vi "TimeShifting.vi"() -> ()   [LabVIEW 2014]
panel:
  in  "Boolean":bool
  out "mag[e^-jwn0.X(w)]":cluster{"-pi to pi":dbl[], dbl[]}(graph)
  out "mag[DTFT{x(n-n0)}]":cluster{"-pi to pi":dbl[], "DTFT op":dbl[]}(graph)
  out "x(n-n0)":dbl[](graph)
  out "x(n)":dbl[](graph)
  out "e^-jwn0.X(w)":cluster{"-pi to pi":dbl[], dbl[]}(graph)
  out "DTFT{x(n-n0)}":cluster{"-pi to pi":dbl[], "DTFT op":dbl[]}(graph)
  out "DTFT{x(n-n0)}":cdb[](array[numeric])
  out "X(w).e^-jwn0":cdb[](array[numeric])
  out "x(n-n0)":dbl[](array[numeric])
  in  "n0":dbl
  out "X(w)":cdb[](array[numeric])
  in  "x(n)":dbl[](array[numeric])
  out "mag response":dbl[](array[numeric])
  # "Instructions"
  # "if\nDTFT{x(n)} ----> X(w)\nthen\nDTFT{x(n-n0)} ----> e^-jwn0.X(w)"
  # "1. enter the input sequence x(n) as array\n2. enter the value by which the time is to be shifted(n>0)\n3. check the input sequence after time shifting\n4. compare the graphs to verify with the property"
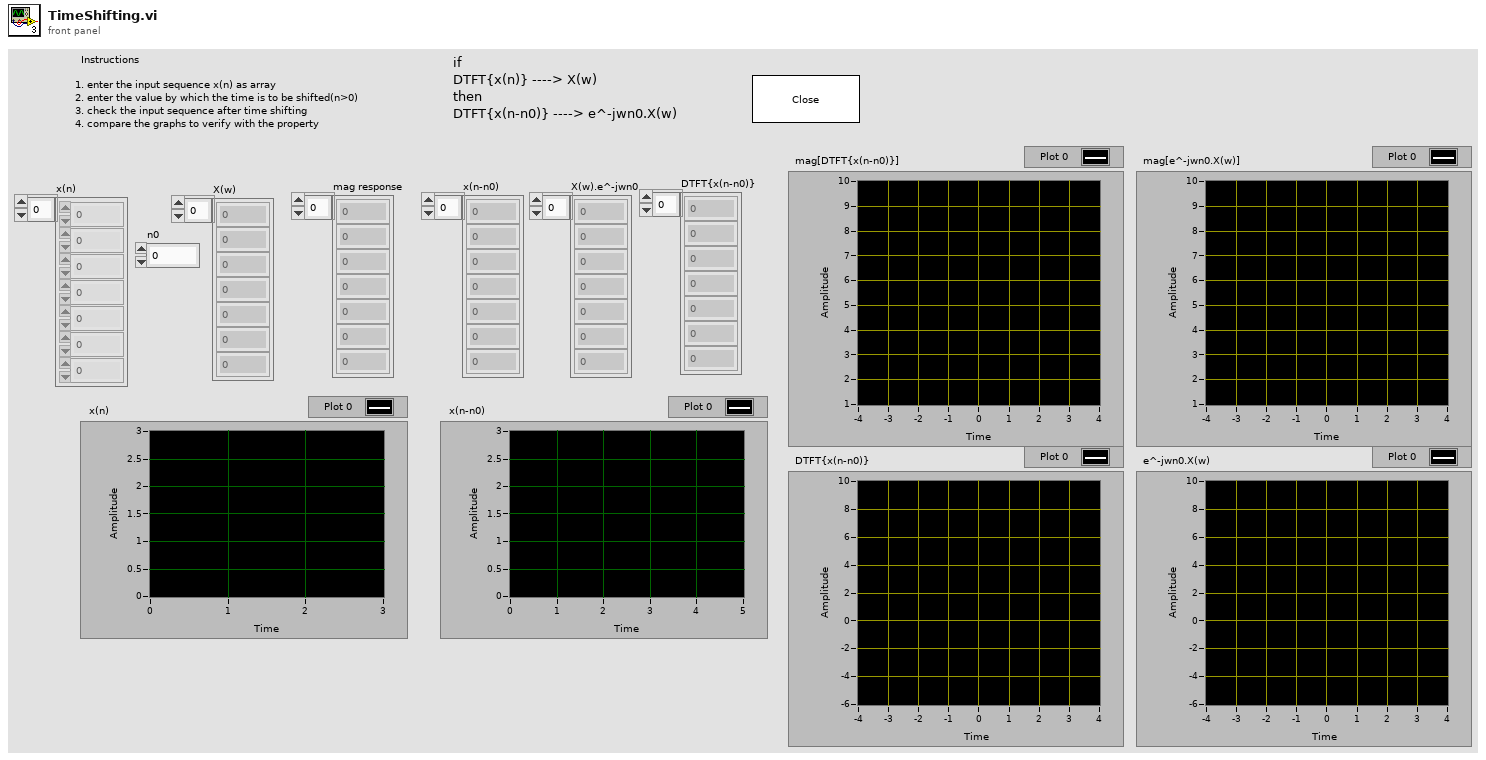
[diagram p1: front panel]
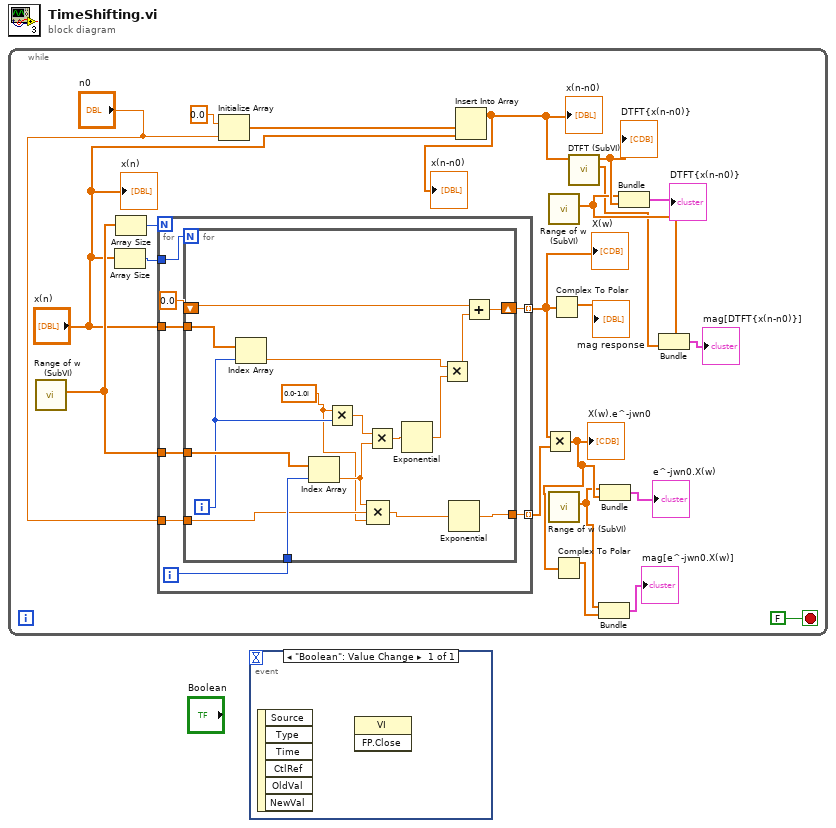
[diagram p0: block diagram]
diagram:
  n1 = while {
    stop <- FALSE stop-if-true
    n2 = call "Range of w (SubVI).vi"() -> ("-pi to pi"=w20:dbl[])  [unwired: 11 in]
    n3 = Array Size(array="x(n)") -> (size(s)=w21:i32)
    n4 = Array Size(array=w20) -> (size(s)=w19:i32)
    n5 = for {
      N: w19 -> [_]
      tunnel: w20 -> [w29]
      tunnel: w21 -> [w28]
      tunnel: "x(n)" -> [w26]
      tunnel: [w25] -> w18 mode=indexing
      tunnel: "n0" -> [w24]
      tunnel: [w23] -> w17 mode=indexing
      i -> [w30]
      n6 = for {
        N: w28 -> [_]
        tunnel: w30 -> [w46]
        tunnel: w29 -> [w45]
        shift-right: [w40] -> w25
        shift-left: 0.0 -> [w39]
        tunnel: w26 -> [w36]
        tunnel: w24 -> [w34]
        tunnel: [w33] -> w23
        i -> [w37]
        w32 = cdb 0.0-1.0i ("x")
        n7 = Index Array(array=w36, index=w37) -> (element=w38:dbl)
        n8 = Index Array(array=w45, index=w46) -> (element=w35:dbl)
        n9 = Multiply(x=w32, y=w37) -> (x*y=w44:cdb)
        n10 = Multiply(x=w44, y=w35) -> (x*y=w43:cdb)
        n11 = Compound Arithmetic op=MULTIPLY(w35, w34, w32) -> (w31:cdb)
        n12 = Exponential(1:w43) -> (0:w42:cdb)
        n13 = Multiply(x=w38, y=w42) -> (x*y=w41:cdb)
        n14 = Exponential(1:w31) -> (0:w33:cdb)
        n15 = Add(x=w39, y=w41) -> (x+y=w40:cdb)
      }
    }
    "X(w)" <- w18
    n16 = Initialize Array(0.0 ("element"), "n0") -> (w11:dbl[])
    n17 = Insert Into Array(array=w11, new element="x(n)") -> (w9:dbl[])  [unwired: 1 in]
    "x(n-n0)" <- w9
    "x(n-n0)" <- w9
    n18 = Multiply(x=w18, y=w17) -> (x*y=w8:cdb[])
    "X(w).e^-jwn0" <- w8
    n19 = call "Range of w (SubVI).vi"() -> ("-pi to pi"=w4:dbl[])  [unwired: 11 in]
    n20 = call "Range of w (SubVI).vi"() -> ("-pi to pi"=w5:dbl[])  [unwired: 11 in]
    n21 = Complex To Polar(r * e^(i*theta)=w18) -> (r=→"mag response":dbl[])  [unwired: 1 out]
    n22 = Complex To Polar(r * e^(i*theta)=w8) -> (r=w7:dbl[])  [unwired: 1 out]
    n23 = call "DTFT (SubVI).vi"("ip array"=w9) -> ("Magnitude op"=w3:dbl[], "DTFT op"=w16:cdb[])  [unwired: 9 in]
    "DTFT{x(n-n0)}" <- w16
    n24 = Bundle("-pi to pi"=w5, w7) -> (→"mag[e^-jwn0.X(w)]":cluster{"-pi to pi":dbl[], dbl[]})  [unwired: 1 in]
    n25 = Bundle("-pi to pi"=w5, w8) -> (→"e^-jwn0.X(w)":cluster{"-pi to pi":dbl[], cdb[]})  [unwired: 1 in]
    n26 = Bundle("-pi to pi"=w4, "DTFT op"=w16) -> (→"DTFT{x(n-n0)}":cluster{"-pi to pi":dbl[], "DTFT op":cdb[]})  [unwired: 1 in]
    n27 = Bundle("-pi to pi"=w4, "Magnitude op"=w3) -> (→"mag[DTFT{x(n-n0)}]":cluster{"-pi to pi":dbl[], "Magnitude op":dbl[]})  [unwired: 1 in]
    "x(n)" <- "x(n)"
  }
  n28 = event shown="[0] \"Boolean\": Value Change" {
    selector: _ -> [_]
    dyn-events: _ -> [_]
    timeout: _ -> [_]
    event "Boolean": Value Change {
      n29 = event-data() -> ()  [unwired: 1 in, 6 out]
      n30 = invoke class="VI" method="FP.Close"() -> ()  [unwired: 3 in, 3 out]
    }
  }
